vi "Acceleration.vi"() -> ()   [LabVIEW 2020]
uses:
  <vilib>/xnet/xnet.llb/XNET Read (Signal Single-point).vi
  <vilib>/xnet/xnet.llb/XNET Create Session (Signal Input Single-point).vi
  SubVI/PlotGraph.llb/GraphPlot.lvlib
  SubVI/PlotGraph.llb/Plot_Y_Graph(RelativeTime-Scope).vi
panel:
  out "AccData":T1
  in  "stop":bool
  out "Channel2_Graph":cluster{dbl[], dbl[]}[](graph)
  out "Channel1_Graph":cluster{dbl[], dbl[]}[](graph)
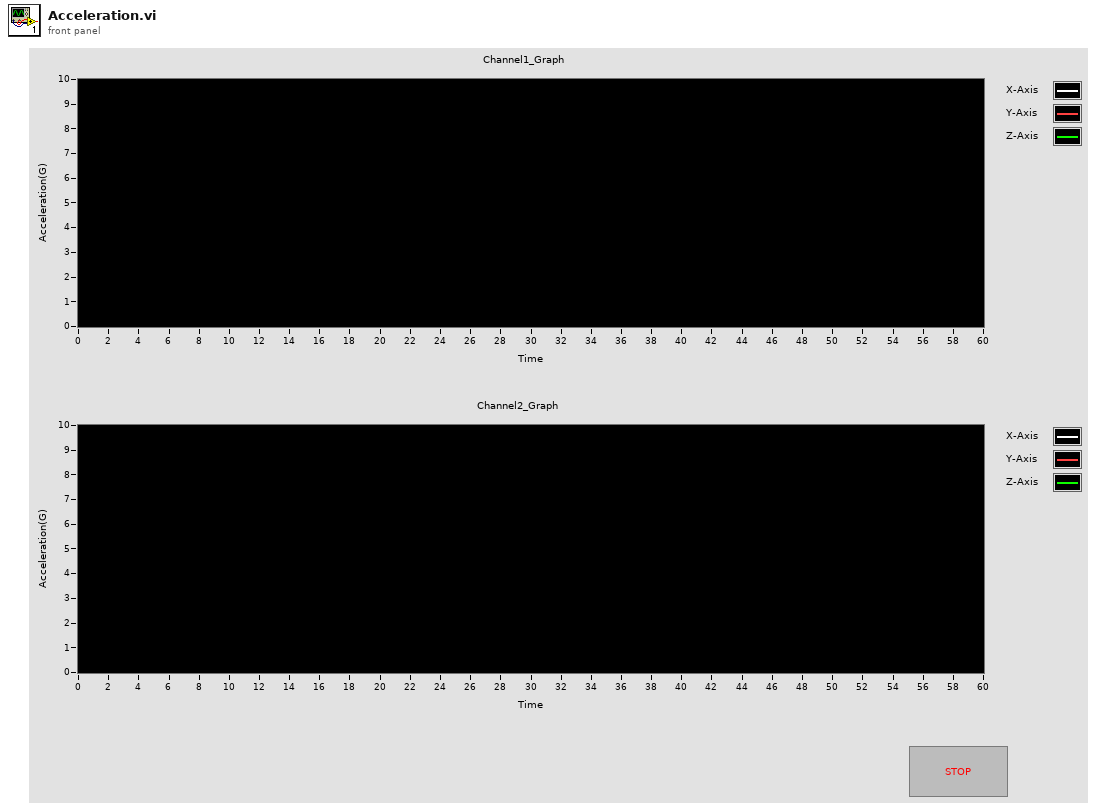
[diagram p1: front panel]
types:
  T1 = cluster{"Ch1_X-Axis(G)":dbl, "Ch1_Y-Axis(G)":dbl, "Ch1_Z-Axis(G)":dbl, "Ch2_X-Axis(G)":dbl, "Ch2_Y-Axis(G)":dbl, "Ch2_Z-Axis(G)":dbl}
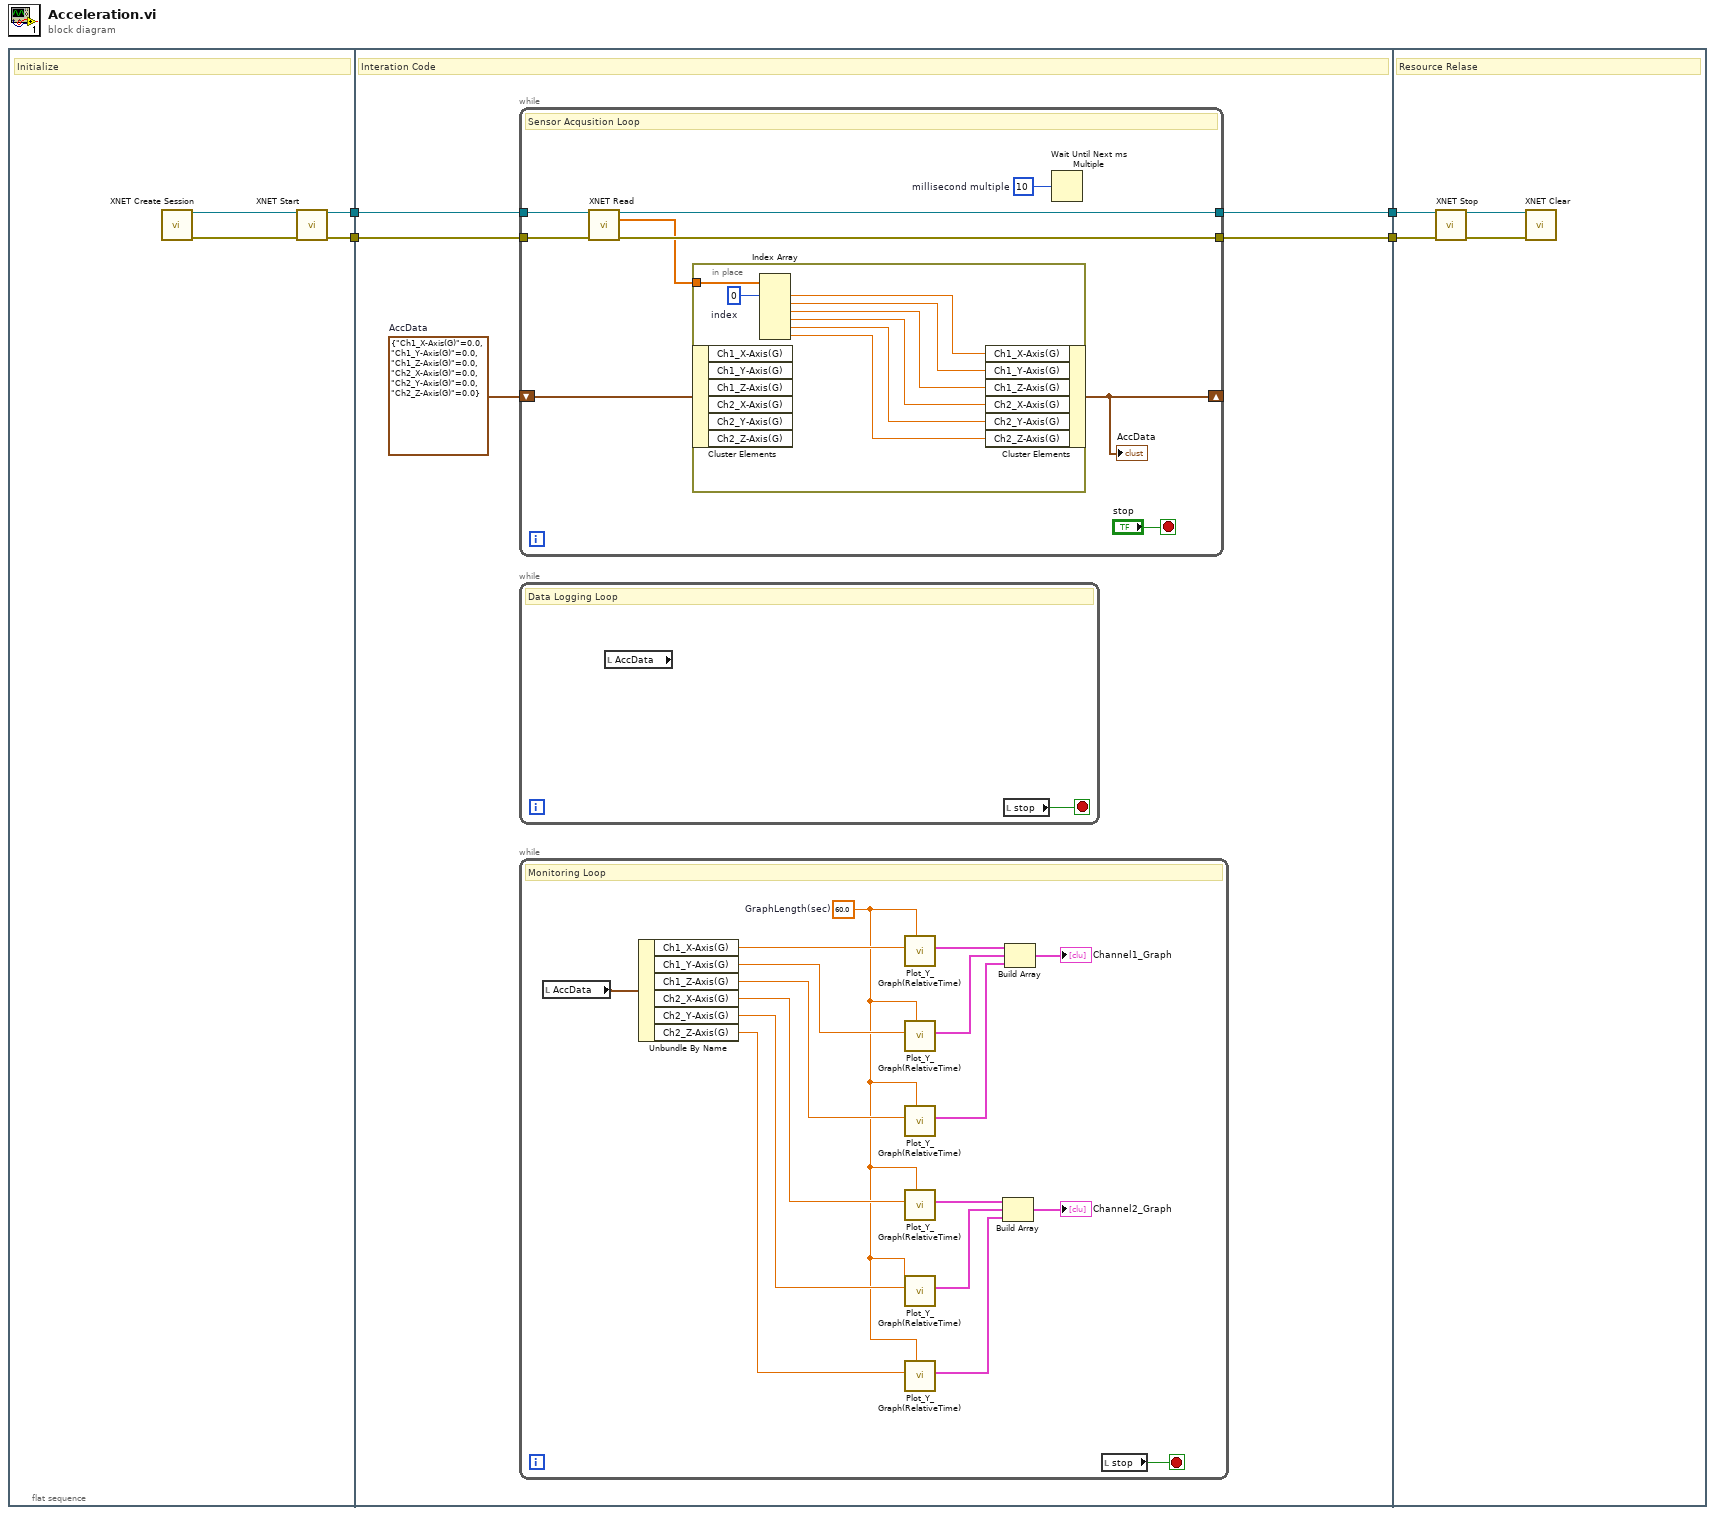
[diagram p0: block diagram]
diagram:
  n1 = flat-sequence {
    tunnel: [w6] -> w4
    tunnel: [w5] -> w3
    tunnel: w4 -> [w13]
    tunnel: w3 -> [w12]
    tunnel: [w11] -> w2
    tunnel: [w10] -> w1
    tunnel: w2 -> [w52]
    tunnel: w1 -> [w51]
    frame #0 {
      # "Initialize"
      n2 = call-poly <vilib>:"XNET Create Session.vi"() -> ("session out"=w8:refnum<k21>, "error out"=w7:errorcluster)  [unwired: 14 in]
      n3 = call <vilib>:"XNET Start.vi"("session in"=w8, "error in (no error)"=w7) -> ("session out"=w6:refnum<k21>, "error out"=w5:errorcluster)  [unwired: 12 in]
    }
    frame #1 {
      w9 = T1 {"Ch1_X-Axis(G)"=0.0, "Ch1_Y-Axis(G)"=0.0, "Ch1_Z-Axis(G)"=0.0, "Ch2_X-Axis(G)"=0.0, "Ch2_Y-Axis(G)"=0.0, "Ch2_Z-Axis(G)"=0.0}  # AccData
      # "Interation Code"
      n4 = while {
        tunnel: w13 -> [w39]
        tunnel: w12 -> [w38]
        tunnel: [w37] -> w11
        tunnel: [w36] -> w10
        shift-right: [w34] -> _
        shift-left: w9 -> [w35]
        stop <- "stop" stop-if-true
        w32 = u32 10  # millisecond multiple
        # "Sensor Acqusition Loop"
        n5 = call-poly <vilib>:"XNET Read.vi"("session in"=w39, "error in (no error)"=w38) -> ("session out"=w36:refnum<k21>, "data"=w33:dbl[], "error out"=w37:errorcluster)  [unwired: 11 in]
        n6 = in-place {
          in-place-border: w33 -> [w48]
          w47 = 0  # index
          n7 = in-place-cluster #1(w35) -> ()  [unwired: 6 out]
          n8 = Index Array(array=w48, index #1=w47) -> (element #1=w46:dbl, element #2=w45:dbl, element #3=w44:dbl, element #4=w43:dbl, element #5=w42:dbl, element #6=w41:dbl)  [unwired: 5 in]
          n9 = in-place-cluster #1("Ch1_X-Axis(G)"=w46, "Ch1_Y-Axis(G)"=w45, "Ch1_Z-Axis(G)"=w44, "Ch2_X-Axis(G)"=w43, "Ch2_Y-Axis(G)"=w42, "Ch2_Z-Axis(G)"=w41) -> (w34:T1)
        }
        "AccData" <- w34
        n10 = Wait Until Next ms Multiple(millisecond multiple=w32) -> ()  [unwired: 1 out]
      }
      n11 = while {
        stop <- w31 stop-if-true
        # "Data Logging Loop"
        n12 = local read "AccData"() -> ()  [unwired: 1 out]
        n13 = local read "stop"() -> (w31:bool)
      }
      n14 = while {
        stop <- w14 stop-if-true
        w17 = 60.0  # GraphLength(sec)
        # "Monitoring Loop"
        n15 = local read "AccData"() -> (w30:T1)
        n16 = Unbundle By Name(w30) -> ("Ch1_X-Axis(G)"=w23:dbl, "Ch1_Y-Axis(G)"=w22:dbl, "Ch1_Z-Axis(G)"=w21:dbl, "Ch2_X-Axis(G)"=w20:dbl, "Ch2_Y-Axis(G)"=w19:dbl, "Ch2_Z-Axis(G)"=w18:dbl)
        n17 = call-poly "Plot_Y_Graph(RelativeTime).vi"("GraphLength(sec)"=w17, "DataInput(Y-Value)"=w23) -> ("XYGraph"=w29:cluster{dbl[], dbl[]})  [unwired: 9 in]
        n18 = call-poly "Plot_Y_Graph(RelativeTime).vi"("GraphLength(sec)"=w17, "DataInput(Y-Value)"=w22) -> ("XYGraph"=w28:cluster{dbl[], dbl[]})  [unwired: 9 in]
        n19 = call-poly "Plot_Y_Graph(RelativeTime).vi"("GraphLength(sec)"=w17, "DataInput(Y-Value)"=w21) -> ("XYGraph"=w27:cluster{dbl[], dbl[]})  [unwired: 9 in]
        n20 = call-poly "Plot_Y_Graph(RelativeTime).vi"("GraphLength(sec)"=w17, "DataInput(Y-Value)"=w20) -> ("XYGraph"=w26:cluster{dbl[], dbl[]})  [unwired: 9 in]
        n21 = call-poly "Plot_Y_Graph(RelativeTime).vi"("GraphLength(sec)"=w17, "DataInput(Y-Value)"=w19) -> ("XYGraph"=w25:cluster{dbl[], dbl[]})  [unwired: 9 in]
        n22 = call-poly "Plot_Y_Graph(RelativeTime).vi"("GraphLength(sec)"=w17, "DataInput(Y-Value)"=w18) -> ("XYGraph"=w24:cluster{dbl[], dbl[]})  [unwired: 9 in]
        n23 = Build Array(w26, w25, w24) -> (→"Channel2_Graph":cluster{dbl[], dbl[]}[])
        n24 = Build Array(w29, w28, w27) -> (→"Channel1_Graph":cluster{dbl[], dbl[]}[])
        n25 = local read "stop"() -> (w14:bool)
      }
    }
    frame #2 {
      # "Resource Relase"
      n26 = call <vilib>:"XNET Stop.vi"("session in"=w51, "error in (no error)"=w52) -> ("session out"=w49:refnum<k21>, "error out"=w50:errorcluster)  [unwired: 12 in]
      n27 = call <vilib>:"XNET Clear.vi"("session in"=w49, "error in (no error)"=w50) -> ()  [unwired: 13 in, 1 out]
    }
  }
